vi "Mod_OFDM_Sliding Correlator.vi"(0 "complex waveform Down Sampled":T1 {"Y" format="%.3f"; "dt" format="%^.2e"; "t0" format="%.4f"}, 2 "Complex Signal Generated":cdb[](array[numeric]), 11 "error in (no error)":errorcluster) -> (4 "complex waveform Down Sampled":T1 {"Y" format="%.3f"; "dt" format="%^.2e"; "t0" format="%.4f"}, 6 "Offset":i32, 15 "error out":errorcluster)   [LabVIEW 2010]
uses:
  <vilib>/addons/Modulation/Analog/controls/Complex Data Waveform.ctl
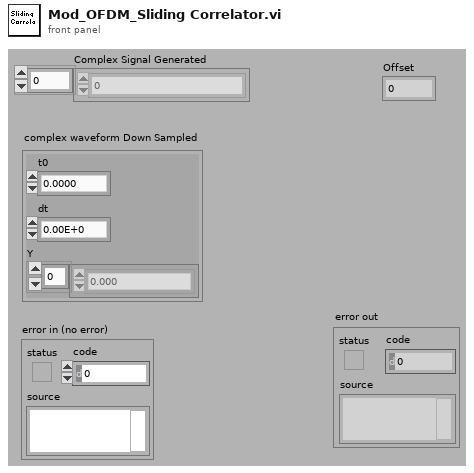
[diagram p1: front panel]
types:
  T1 = typedef "Complex Data Waveform.ctl" = cluster{"t0":dbl, "dt":dbl, "Y":cdb[]}
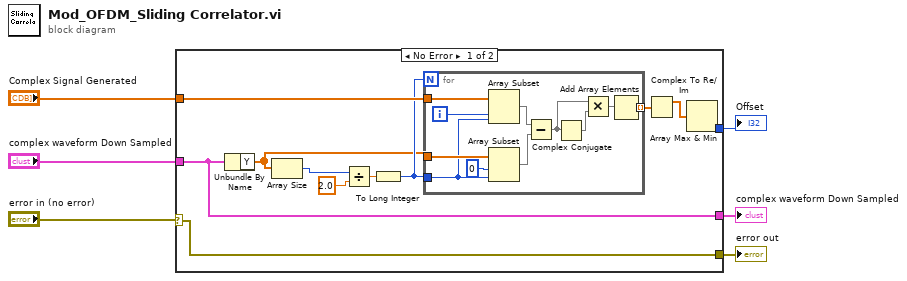
[diagram p0: block diagram]
diagram:
  n1 = case shown="No Error" "error in (no error)" {
    selector: "error in (no error)" -> [w8 w29]
    tunnel: "Complex Signal Generated" -> [w17 _]
    tunnel: [w14 _] -> w5
    tunnel: "complex waveform Down Sampled" -> [w7 _]
    tunnel: [w8 w29] -> w3
    tunnel: [w7 _] -> w1
    frame No Error {
      n2 = Unbundle By Name(w7) -> ("Y"=w9:cdb[])
      n3 = Array Size(array=w9) -> (size(s)=w13:i32)
      n4 = Divide(x=w13, y=2.0) -> (x/y=w11:dbl)
      n5 = To Long Integer(number=w11) -> (32bit integer=w10:i32)
      n6 = for {
        N: w10 -> [_]
        tunnel: w9 -> [w27]
        tunnel: w17 -> [w26]
        tunnel: [w19] -> w16 mode=indexing
        tunnel: w10 -> [w18]
        i -> [w25]
        n7 = Array Subset(array=w26, index=w25, length=w18) -> (w24:cdb[])
        n8 = Array Subset(array=w27, index=0, length=w18) -> (w23:cdb[])
        n9 = Subtract(x=w24, y=w23) -> (x-y=w21:cdb[])
        n10 = Complex Conjugate(1:w21) -> (0:w22:cdb[])
        n11 = Multiply(x=w21, y=w22) -> (x*y=w20:cdb[])
        n12 = Add Array Elements(numeric array=w20) -> (sum=w19:cdb)
      }
      n13 = Complex To Re/Im(x + iy=w16) -> (x=w15:dbl[])  [unwired: 1 out]
      n14 = Array Max & Min(array=w15) -> (min index (indices)=w14:i32)  [unwired: 3 out]
    }
    frame Error {
    }
  }
  "Offset" <- w5
  "error out" <- w3
  "complex waveform Down Sampled" <- w1
